vi "New Task.vi"(4 "BuildSpec Type":string, 6 "Target":string, 7 "Task in":refnum<class "Task.lvclass">, 8 "error in (no error)":errorcluster, 9 "BuildSpec Name":string, 10 "ProjectPath":path, 11 "Name":string) -> (0 "error out":errorcluster, 3 "Task out":refnum<class "Task.lvclass">)   [LabVIEW 2017, in "Task Interface.lvlib" / "Task.lvclass"]
uses:
  Task.lvclass
  Status.ctl
  Task.lvclass/Task.ctl
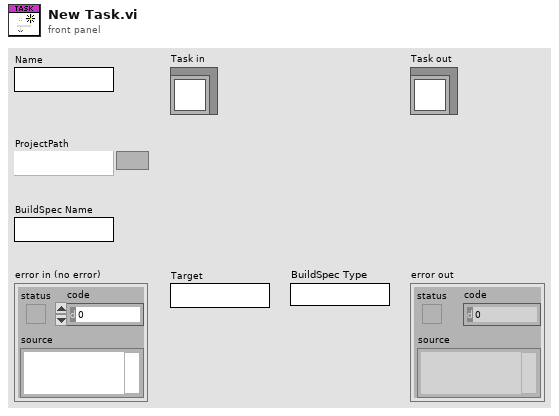
[diagram p1: front panel]
types:
  T1 = typedef "Task Interface.lvlib/Task.lvclass/Status.ctl" = enum16{"Created", "Added", "Pending", "Queued", "Processing", "Cleaning", "Building", "Finished", "Failed", "Removed", "Not found"}
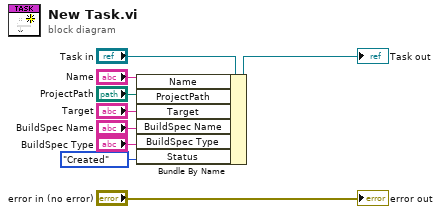
[diagram p0: block diagram]
diagram:
  n1 = Bundle By Name(cluster="Task in", "Name"="Name", "ProjectPath"="ProjectPath", "Target"="Target", "BuildSpec Name"="BuildSpec Name", "BuildSpec Type"="BuildSpec Type", "Status"=Status."Created") -> (→"Task out":refnum<class "Task.lvclass">)
  "error out" <- "error in (no error)"
